vi "getdonneestacheuser.vi"(1 "id":dbl, 2 "Fichier DB":string) -> (0 "Données tache user":string[][](table))   [LabVIEW 2024]
uses:
  <vilib>/drjdpowell/SQLite Library/SQL Connection/Connection.lvclass
  <vilib>/drjdpowell/SQLite Library/SQL Connection/Open (string).vi
  <vilib>/drjdpowell/SQLite Library/SQLite.lvlib
  <vilib>/drjdpowell/SQLite Library/SQL Connection/Execute SQL.vi
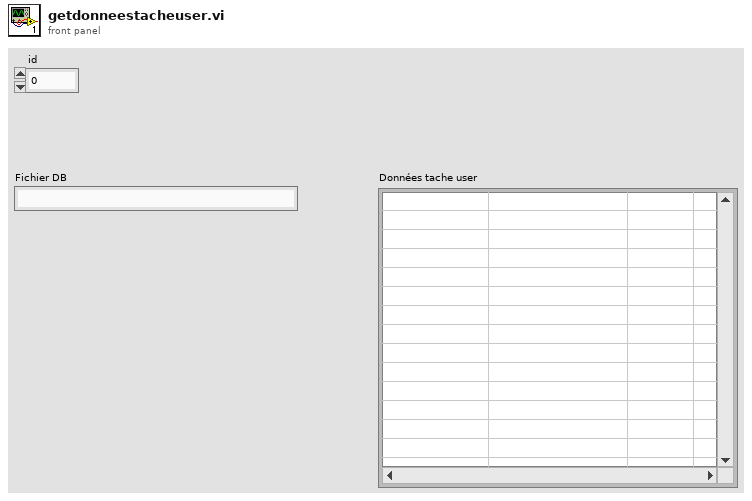
[diagram p1: front panel]
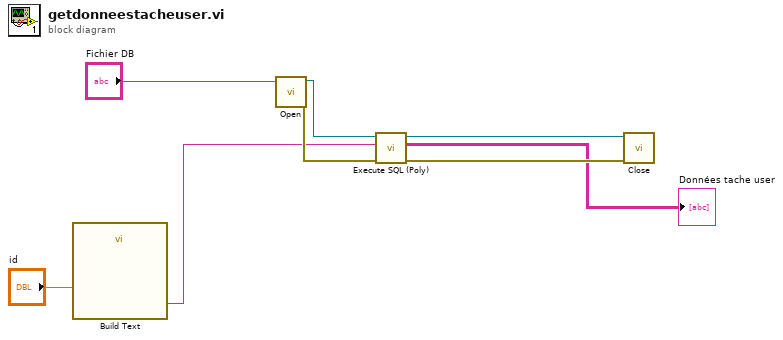
[diagram p0: block diagram]
diagram:
  n1 = call "Build Text"("id"="id") -> ("Result"=w2:string)  [unwired: 13 in, 1 out]
  n2 = call-poly <vilib>:"Open.vi"("db file"="Fichier DB") -> ("error out"=w4:errorcluster, "SQLite Connection"=w5:refnum<class "Connection.lvclass">)  [unwired: 9 in]
  n3 = call-poly <vilib>:"Execute SQL (Poly).vi"("error in (no error)"=w4, "SQL"=w2, "SQLite Connection in"=w5) -> ("error out"=w7:errorcluster, "Result Set"=→"Données tache user":string[][], "SQLite Connection"=w8:refnum<class "Connection.lvclass">)  [unwired: 5 in, 1 out]
  n4 = call-dynamic "Close.vi"("error in (no error)"=w7, "SQLite Connection in"=w8) -> ()  [unwired: 9 in, 1 out]
